vi "Servo Example.vi"() -> ()   [LabVIEW 2013, in "LabVIEW Interface for Arduino.lvlib"]
doc: "An example using two servos with the LabVIEW Interface for Arduino."
uses:
  <vilib>/LabVIEW Interface for Arduino/LabVIEW Interface for Arduino.lvlib
panel:
  in  "Press Button":bool
  in  "Stop":bool
  out "Servo 0":dbl(knob) scale=0.0..180.0
  in  "Number of Servos":u8=2
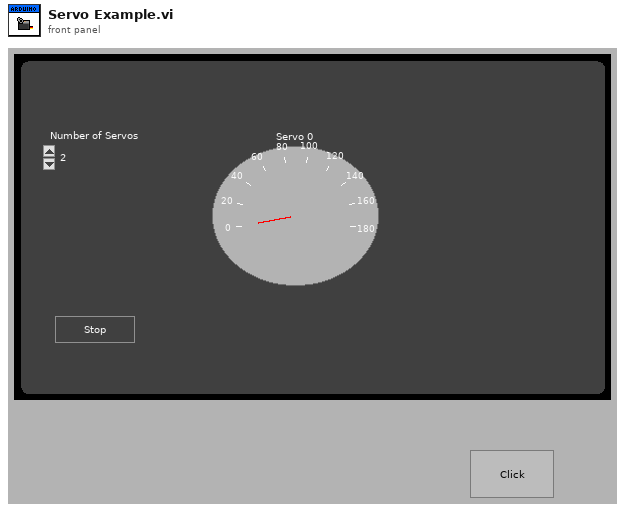
[diagram p1: front panel]
types:
  T1 = typedef "LabVIEW Interface for Arduino.lvlib/Arduino Resource.ctl" = cluster{"VISA resource":refnum<visa-resource-name>, "Board Type":T2, "Connection Type":enum8{"USB / Serial"}, "Bytes Per Packet (15)":u8}
  T2 = typedef "LabVIEW Interface for Arduino.lvlib/Board Type.ctl" = enum16{"Uno", "Dimuelanove w/Atmega 328", "Mega 2560"}
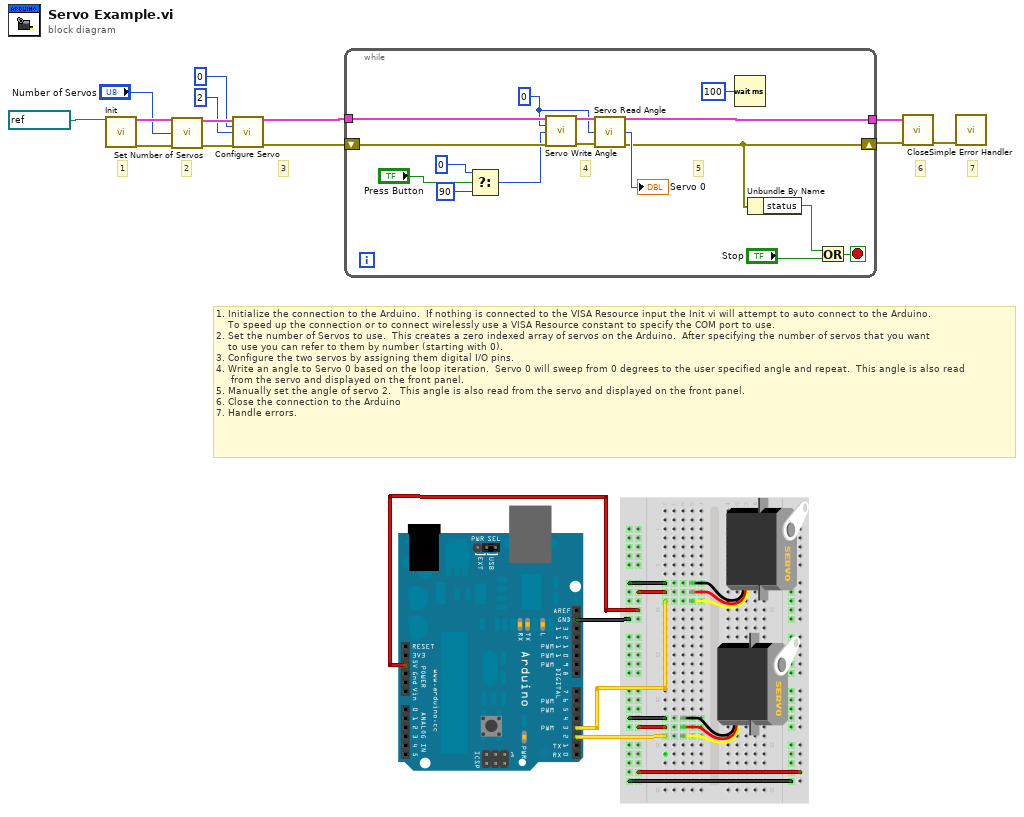
[diagram p0: block diagram]
diagram:
  # "1. Initialize the connection to the Arduino.  If nothing is connected to the VISA Resource input the Init vi will attempt to auto connect to the Arduino.\n    To speed up the connection or to connect wirelessly use a VISA Resource constant to specify the COM port to use.\n2. Set the number of Servos to use.  This creates a zero indexed array of servos on the Arduino.  After specifying the number of servos that you want \n    to use you can refer to them by number (starting with 0).\n3. Configure the two servos by assigning them digital I/O pins.\n4. Write an angle to Servo 0 based on the loop iteration.  Servo 0 will sweep from 0 degrees to the user specified angle and repeat.  This angle is also read\n     from the servo and displayed on the front panel.\n5. Manually set the angle of servo 2.   This angle is also read from the servo and displayed on the front panel.\n6. Close the connection to the Arduino\n7. Handle errors."
  # "7"
  # "6"
  # "3"
  # "2"
  # "1"
  n1 = call <vilib>:"Init.vi"("VISA resource"=refnum<visa-resource-name> "COM3") -> ("Arduino Resource"=w13:T1, "error out"=w12:errorcluster)  [unwired: 17 in]
  n2 = call <vilib>:"Set Number of Servos.vi"("Arduino Resource"=w13, "Number Of Servos (1)"="Number of Servos", "error in"=w12) -> ("Arduino Resource"=w10:T1, "error out"=w9:errorcluster)  [unwired: 11 in]
  n3 = call <vilib>:"Configure Servo.vi"("Arduino Resource"=w10, "Servo Number (0)"=u8 0 ("Servo Number"), "DIO Pin (2)"=u8 2 ("Servo Number"), "error in"=w9) -> ("Arduino Resource"=w2:T1, "error out"=w1:errorcluster)  [unwired: 10 in]
  n4 = while {
    tunnel: w2 -> [w29]
    tunnel: [w20] -> w5
    shift-right: [w19] -> w6
    shift-left: w1 -> [w27]
    stop <- w25 stop-if-true
    w23 = u8 0 ("Servo Number")
    # "5"
    # "4"
    n5 = Select(t=u8 0 ("Servo Number"), s="Press Button", f=u8 90) -> (s? t:f=w16:u8)
    n6 = call <vilib>:"Servo Write Angle.vi"("Arduino Resource"=w29, "Servo Number"=w23, "Angle (Degrees)"=w16, "error in"=w27) -> ("Arduino Resource"=w28:T1, "error out"=w26:errorcluster)  [unwired: 10 in]
    n7 = call <vilib>:"Servo Read Angle.vi"("Arduino Resource"=w28, "Servo Number"=w23, "error in"=w26) -> ("Arduino Resource"=w20:T1, "Angle (Degrees)"=→"Servo 0":u8, "error out"=w19:errorcluster)  [unwired: 10 in]
    n8 = Wait (ms)(milliseconds to wait=u32 100) -> ()  [unwired: 1 out]
    n9 = Unbundle By Name(w19) -> ("status"=w24:bool)
    n10 = Or(x=w24, y="Stop") -> (x .or. y?=w25:bool)
  }
  n11 = call <vilib>:"Close.vi"("Arduino Resource"=w5, "error in"=w6) -> ("error out"=w3:errorcluster)  [unwired: 13 in]
  n12 = call <vilib>:"Simple Error Handler.vi"("error in (no error)"=w3) -> ()  [unwired: 4 in, 5 out]
